vi "DAQ 1SDI v05.1.vi"() -> ()   [LabVIEW 2013]
uses:
  <instrlib>/niScope/Controls/niScope vertical coupling.ctl
  Strict Type Defs/type_meas_enum.ctl
panel:
  in  "stop":bool
  in  "Monitors":enum32{"Monitors On", "Monitors Off"}(tab)
  out "Key rate A|B":dbl(graph)=5.494105801184175
  out "covariance A|B":dbl(graph)=0.0005477195800282943
  out "Conditional variance A|B":dbl(graph)=0.016324687192990704
  out "Loop count":i32=34024
  in  "Settings":enum32{"Settings and Record", "Under the hood"}(tab)
  in  "save or monitor":bool
  in  "File location":path=path "C:/ni-rt/LabVIEW Data/July1/35dB109"
  in  "Type of measurement":T1=enum."electronic"
  in  "File root name":string="Real_9"
  in  "Number of samples save":i32=10000000 format="%.0p"
  in  "reset sn":bool
  in  "Shot noise start":bool
  in  "Additional text":string="OPA 1 optical power set to 15mV on HD A.\nOPA 2 optical power set to 15mV on HD B.\nLocal oscillator is set to 5V on HD.\nParametric gain set to 15 for OPA 1.\nParametric gain set to 15 for OPA 2.\nVertical range set to 0.5V for both channels.\nSample rate set to 14MS/s.\nMax input freq set to7MHz.\nVisibility between OPA 1 & OPA 2 = 99.6\nVisibility between OPA 1 & L.O.B = 98.9\nVisibility between OPA 1 & L.O. A = 98.9\nBoth squeezers expected to produce -7dB/11dB.\nLoss on EPR B =55.33% (3.5dB) \n"
  in  "Record":bool
  in  "Number of Files":i32=2
  out "File count":i32=1
  in  "Monitors On":bool=TRUE
  in  "Number of samples monitor":i32=120000 format="%.0p"
  in  "DAQ Cards":T2={"DAQ Card 1"="Dev2", "DAQ Card 2"="Dev2"}
  in  "Channel parameters":T4(array[cluster])=[{"Channel name"="0", "Input impedance (Ohms)"=2, "Maximum input frequency (Hz)"=7000000.0, "vertical coupling"=1, "Probe attenuation"=1.0, "Vertical range (V)"=0.5, "Vertical offset"=0.0, "channel enabled"=TRUE}, {"Channel name"="1", "Input impedance (Ohms)"=2, "Maximum input frequency (Hz)"=7000000.0, "vertical coupling"=1, "Probe attenuation"=1.0, "Vertical range (V)"=0.5, "Vertical offset"=0.0, "channel enabled"=TRUE}] {"Input impedance (Ohms)" items=["1 mega ohm"=0, "50 ohms"=2]; "Maximum input frequency (Hz)" format="%#_6p"; "vertical coupling" items=["AC", "DC", "Ground"]}
  out "Actual samples acquired ch 0":i32=120000
  out "Actual samples acquired ch 1":i32=120000
  out "Parameters values file":string="PARAMETERS VALUES\r\rTuesday, July 1, 2014\r4:56 PM\r\rMaster ch 0 <-> HD1 AC a-b\nMaster ch 1 <-> HD2 AC a-b\n\rSample rate : \rMaster : 14.285714E+6 Samples per second\rNumber of samples :\rMaster ch 0 : 120.000000E+3\rMaster ch 1 : 120.000000E+3\rFiles names : \rReal_9_electronic_ParametersValues_120000.txt\rReal_9_electronic_mch01_240000.txt\r\rOPA 1 optical power set to 15mV on HD A.\nOPA 2 optical power set to 15mV on HD B.\nLocal oscillator is set to 5V on HD.\nParametric gain set to 15 for OPA 1.\nParametric gain set to 15 for OPA 2.\nVertical range set to 0.5V for both channels.\nSample rate set to 14MS/s.\nMax input freq set to7MHz.\nVisibility between OPA 1 & OPA 2 = 99.6\nVisibility between OPA 1 & L.O.B = 98.9\nVisibility between OPA 1 & L.O. A = 98.9\nBoth squeezers expected to produce -7dB/11dB.\nLoss on EPR B =55.33% (3.5dB) \n"
  in  "IIR filter specifications":T5={"Topology"=enum."Butterworth", "Type"=enum."Bandpass", "Order"=6, "Lower Fc"=2900000.0, "Upper Fc"=3100000.0, "PB Ripple"=1.0, "SB Attenuation"=60.0} {"PB Ripple" format="%0.2f"; "SB Attenuation" format="%0.2f"; "Lower Fc" format="%0.2p"; "Upper Fc" format="%0.2p"}
  out "error out":errorcluster caption="error out final"
  in  "max time (s)":dbl=10.0 caption="Time to run (s)"
  in  "Reference position":dbl(slide)=50.0 scale=0.0..100.0
  in  "Minimum sample rate (S/s)":dbl=14000000.0 format="%#_6p"
  out "Video bandwidth (Hz)":dbl=1.4
  # "Variance won't be displayed until shot noise is taken"
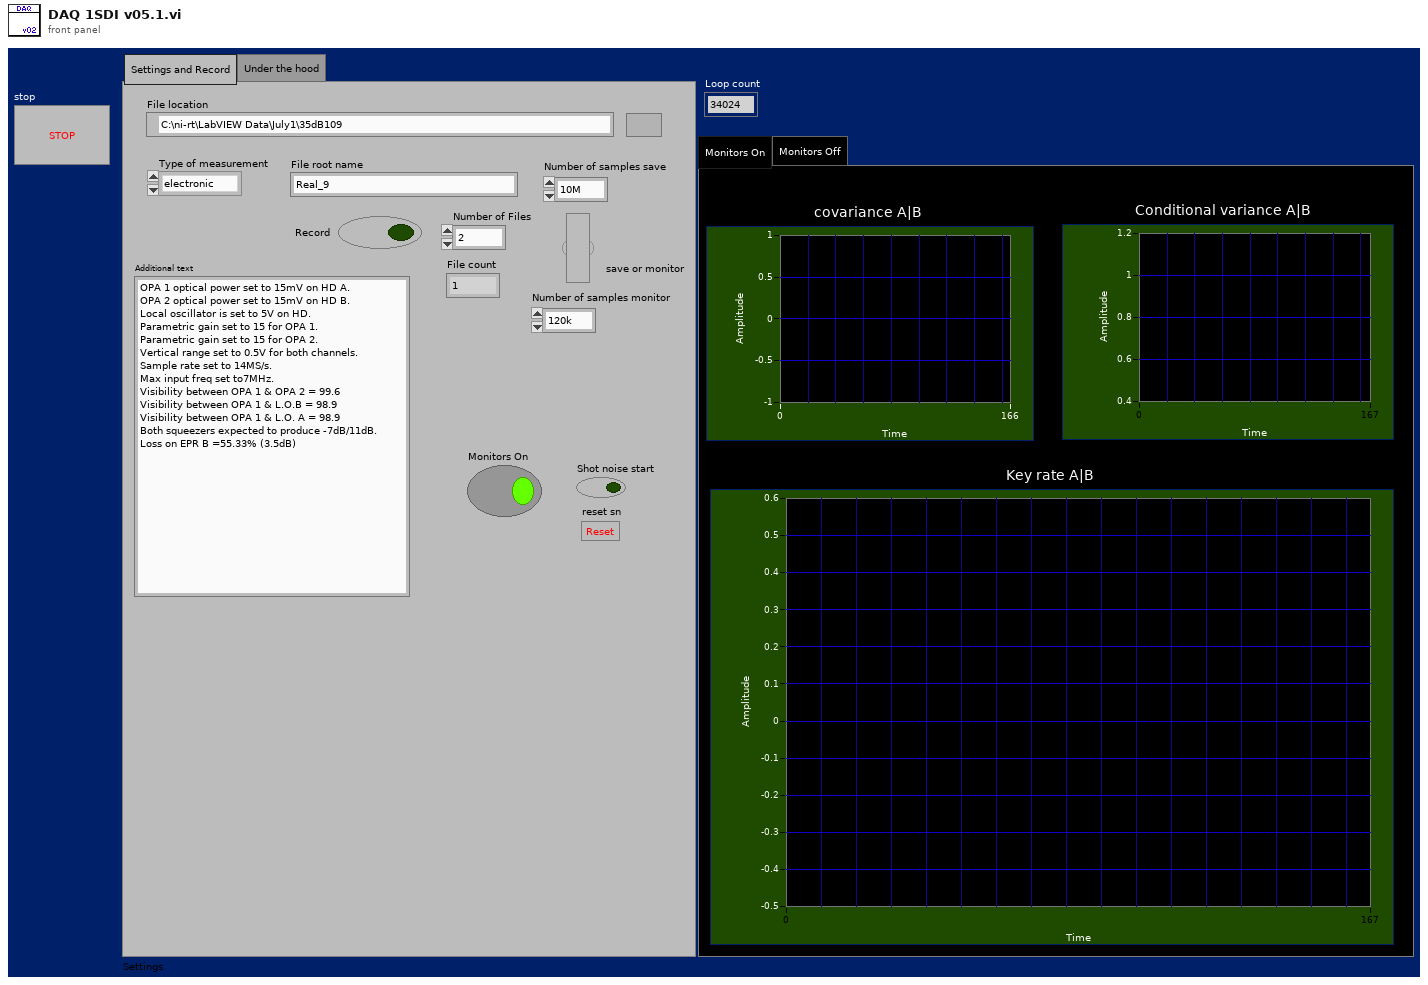
[diagram p1: front panel]
types:
  T1 = typedef "type_meas_enum.ctl" = enum16{"shot", "x", "p", "electronic"}
  T2 = cluster{"DAQ Card 1":refnum<k15>, "DAQ Card 2":refnum<k15>}
  T3 = typedef "niScope vertical coupling.ctl" = i32
  T4 = cluster{"Channel name":string, "Input impedance (Ohms)":u32, "Maximum input frequency (Hz)":dbl, "vertical coupling":T3, "Probe attenuation":dbl, "Vertical range (V)":dbl, "Vertical offset":dbl, "channel enabled":bool}[]
  T5 = cluster{"Topology":enum16{"Off", "Butterworth", "Chebyshev", "Inverse Chebyshev", "Elliptic", "Bessel"}, "Type":enum16{"Lowpass", "Highpass", "Bandpass", "Bandstop"}, "Order":i32, "Lower Fc":dbl, "Upper Fc":dbl, "PB Ripple":dbl, "SB Attenuation":dbl}
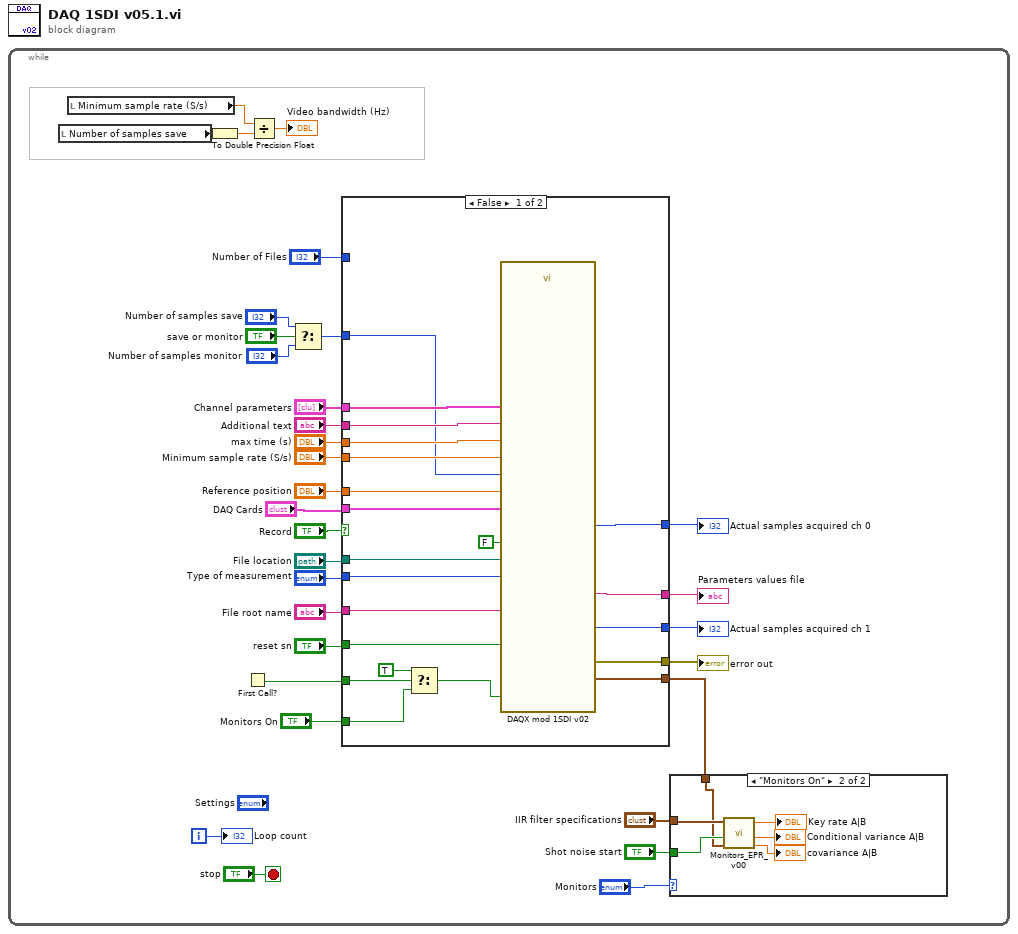
[diagram p0: block diagram]
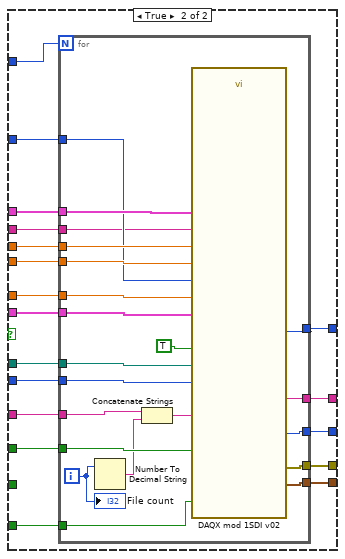
[diagram p2: hidden frame]
diagram:
  n1 = while {
    i -> [w18]
    stop <- "stop" stop-if-true
    n2 = local read "Number of samples save"() -> (w32:i32)
    n3 = local read "Minimum sample rate (S/s)"() -> (w30:dbl)
    n4 = To Double Precision Float(number=w32) -> (double precision float=w29:dbl)
    n5 = First Call?() -> (First Call?: T/F=w6:bool)
    n6 = Divide(x=w30, y=w29) -> (x/y=→"Video bandwidth (Hz)":dbl)
    n7 = Select(t="Number of samples save", s="save or monitor", f="Number of samples monitor") -> (s? t:f=w3:i32)
    n8 = case shown="False" "Record" {
      tunnel: "Channel parameters" -> [w52 w71]
      tunnel: "max time (s)" -> [w50 w70]
      tunnel: "Minimum sample rate (S/s)" -> [w49 w69]
      tunnel: "Reference position" -> [w47 w68]
      tunnel: w3 -> [w48 w67]
      tunnel: [w41 w66] -> w24
      tunnel: "DAQ Cards" -> [w46 w65]
      tunnel: "File location" -> [w45 w64]
      tunnel: "Type of measurement" -> [w44 w63]
      tunnel: [w40 w62] -> w21
      tunnel: "File root name" -> [w42 w61]
      tunnel: [w39 w60] -> w19
      tunnel: [w38 w59] -> w17
      tunnel: [w33 w58] -> w16
      tunnel: "reset sn" -> [w43 w57]
      tunnel: "Additional text" -> [w51 w56]
      tunnel: "Number of Files" -> [_ w55]
      tunnel: "Monitors On" -> [w36 w54]
      tunnel: w6 -> [w37 _]
      frame False {
        n9 = Select(t=TRUE, s=w37, f=w36) -> (s? t:f=w34:bool)
        n10 = call "DAQX mod 1SDI v02.vi"("resource names"=w46, "Record Data"=FALSE, "numSamples"=w48, "max time (s)"=w50, "min sample rate"=w49, "File location"=w45, "reference position"=w47, "Additional text"=w51, "Type of measurement"=w44, "Name root"=w42, "Monitor On"=w34, "channel parameters"=w52, "reset sn"=w43) -> ("wfm out 1"=w33:waveform(dbl)[], "Parameters values file"=w40:string, "actualSamples 2"=w41:i32, "actualSamples 3"=w39:i32, "error out 2"=w38:errorcluster)  [unwired: 8 in, 2 out]
      }
      frame True {
        n11 = for {
          N: w55 -> [_]
          tunnel: w71 -> [w92]
          tunnel: w70 -> [w91]
          tunnel: w69 -> [w90]
          tunnel: w68 -> [w89]
          tunnel: w67 -> [w88]
          tunnel: [w87] -> w66
          tunnel: w65 -> [w86]
          tunnel: w64 -> [w85]
          tunnel: w63 -> [w84]
          tunnel: [w83] -> w62
          tunnel: w61 -> [w76]
          tunnel: [w82] -> w60
          tunnel: [w81] -> w59
          tunnel: [w80] -> w58
          tunnel: w57 -> [w79]
          tunnel: w56 -> [w78]
          tunnel: w54 -> [w72]
          i -> [w73]
          n12 = Number To Decimal String(number=w73) -> (decimal integer string=w74:string)  [unwired: 1 in]
          n13 = Concatenate Strings(w76, w74) -> (w75:string)
          n14 = call "DAQX mod 1SDI v02.vi"("resource names"=w86, "Record Data"=TRUE, "numSamples"=w88, "max time (s)"=w91, "min sample rate"=w90, "File location"=w85, "reference position"=w89, "Additional text"=w78, "Type of measurement"=w84, "Name root"=w75, "Monitor On"=w72, "channel parameters"=w92, "reset sn"=w79) -> ("wfm out 2"=w80:waveform(dbl)[], "Parameters values file"=w83:string, "actualSamples 2"=w87:i32, "actualSamples 3"=w82:i32, "error out 2"=w81:errorcluster)  [unwired: 8 in, 2 out]
          "File count" <- w73
        }
      }
    }
    "Actual samples acquired ch 0" <- w24
    "Parameters values file" <- w21
    "Actual samples acquired ch 1" <- w19
    "error out" <- w17
    n15 = case shown="\"Monitors On\"" "Monitors" {
      tunnel: w16 -> [_ w93]
      tunnel: "IIR filter specifications" -> [_ w95]
      tunnel: "Shot noise start" -> [_ w94]
      frame "Monitors Off" {
      }
      frame "Monitors On" {
        n16 = call "Monitors_EPR_v00.vi"("wfm"=w93, "Shot noise start"=w94, "IIR filter specifications"=w95) -> ("covariance"=→"covariance A|B":dbl, "conditional variance A|B"=→"Conditional variance A|B":dbl, "Key Rate A|B"=→"Key rate A|B":dbl)  [unwired: 6 in]
      }
    }
    "Loop count" <- w18
  }
